vi "Read dEL_ArcsPS.vi"(8 "error in (no error)":errorcluster, 11 "DifftrackAzEl in":refnum<class "DifftrackAzEl.lvclass">) -> (0 "error out":errorcluster, 2 "dEL_ArcsPS":dbl[unit] min=-4.84813681109536e-05 max=4.84813681109536e-05, 3 "DifftrackAzEl out":refnum<class "DifftrackAzEl.lvclass">)   [LabVIEW 2014, in "TCSDataDefinitions.lvlib" / "TCSCommand.lvlib" / "TargetConfiguration.lvlib" / "Target.lvlib" / "DifftrackAzEl.lvclass"]
uses:
  DifftrackAzEl.lvclass
  DifftrackAzEl.lvclass/DifftrackAzEl.ctl
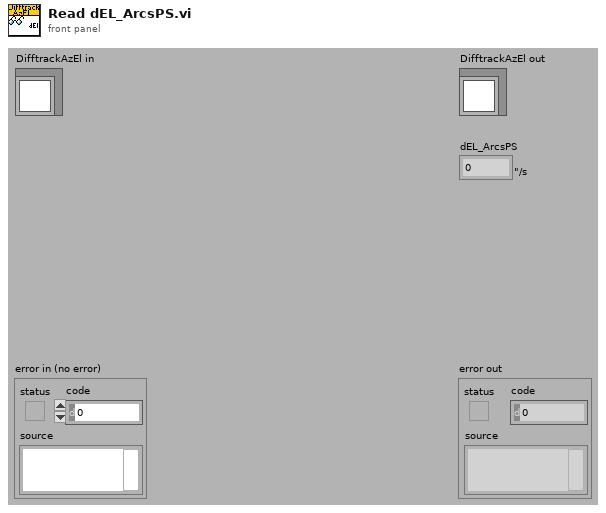
[diagram p1: front panel]
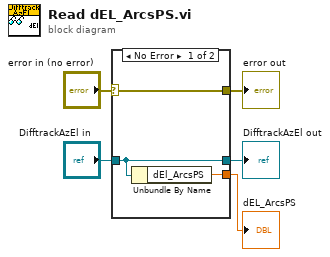
[diagram p0: block diagram]
diagram:
  n1 = case shown="No Error" "error in (no error)" {
    selector: "error in (no error)" -> [w8 w9]
    tunnel: [w8 w9] -> w4
    tunnel: [w7 w10] -> w2
    tunnel: "DifftrackAzEl in" -> [w7 w10]
    tunnel: [w6 _] -> w1
    frame No Error {
      n2 = Unbundle By Name(w7) -> ("dEl_ArcsPS"=w6:dbl[unit])
    }
    frame Error {
    }
  }
  "error out" <- w4
  "DifftrackAzEl out" <- w2
  "dEL_ArcsPS" <- w1
